vi "Untitled 5 (SubVI).vi"(11 "Button":u16) -> (3 "new picture":picture)   [LabVIEW 2020]
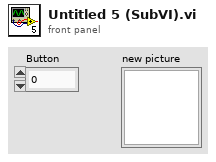
[diagram p1: front panel]
types:
  T1 = cluster{"dimension size":i32, "dimension size":i32, "dimension size":i32, "dimension size":i32}
  T2 = cluster{"dimension size":i32, "dimension size":i32}
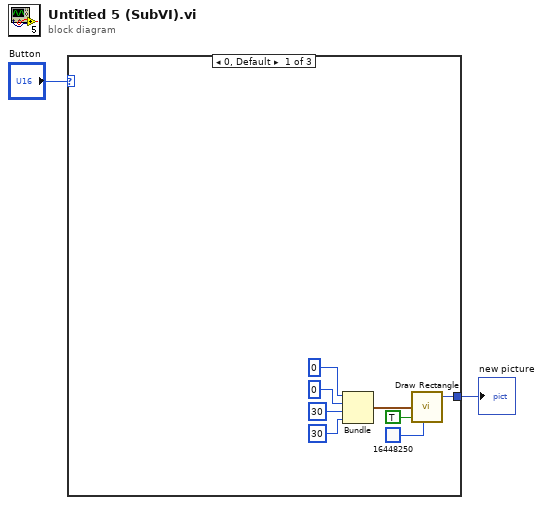
[diagram p0: block diagram]
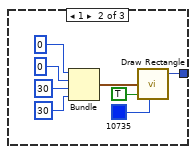
[diagram p2: hidden frame]
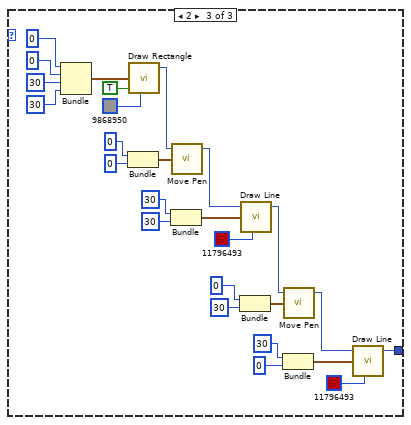
[diagram p3: hidden frame]
diagram:
  n1 = case shown="0, Default" "Button" {
    tunnel: [w3 w11 w19] -> w1
    frame 0, Default {
      n2 = Bundle("dimension size"=0, "dimension size"=0, "dimension size"=30, "dimension size"=30) -> (w10:T1)  [unwired: 1 in]
      n3 = call <vilib>:"Draw Rectangle.vi"("rect"=w10, "fill?(F)"=TRUE, "color(black)"=u32 16448250) -> ("new picture"=w3:picture)  [unwired: 6 in]
    }
    frame 1 {
      n4 = Bundle("dimension size"=0, "dimension size"=0, "dimension size"=30, "dimension size"=30) -> (w18:T1)  [unwired: 1 in]
      n5 = call <vilib>:"Draw Rectangle.vi"("rect"=w18, "fill?(F)"=TRUE, "color(black)"=u32 10735) -> ("new picture"=w11:picture)  [unwired: 6 in]
    }
    frame 2 {
      n6 = Bundle("dimension size"=0, "dimension size"=0, "dimension size"=30, "dimension size"=30) -> (w44:T1)  [unwired: 1 in]
      n7 = Bundle("dimension size"=0, "dimension size"=0) -> (w34:T2)  [unwired: 1 in]
      n8 = call <vilib>:"Draw Rectangle.vi"("rect"=w44, "fill?(F)"=TRUE, "color(black)"=u32 9868950) -> ("new picture"=w33:picture)  [unwired: 6 in]
      n9 = Bundle("dimension size"=30, "dimension size"=30) -> (w29:T2)  [unwired: 1 in]
      n10 = call <vilib>:"Move Pen.vi"("new position"=w34, "picture"=w33) -> ("new picture"=w30:picture)  [unwired: 3 in]
      n11 = Bundle("dimension size"=0, "dimension size"=30) -> (w28:T2)  [unwired: 1 in]
      n12 = call <vilib>:"Draw Line.vi"("picture"=w30, "end point"=w29, "color(black)"=u32 11796493) -> ("new picture"=w20:picture)  [unwired: 6 in]
      n13 = Bundle("dimension size"=30, "dimension size"=0) -> (w26:T2)  [unwired: 1 in]
      n14 = call <vilib>:"Move Pen.vi"("new position"=w28, "picture"=w20) -> ("new picture"=w27:picture)  [unwired: 3 in]
      n15 = call <vilib>:"Draw Line.vi"("picture"=w27, "end point"=w26, "color(black)"=u32 11796493) -> ("new picture"=w19:picture)  [unwired: 6 in]
    }
  }
  "new picture" <- w1
